vi "scada.vi"() -> ()   [LabVIEW 2014]
panel:
  in  "?":bool
  out "B7":bool
  out "B6":bool
  out "B5":bool
  out "B4":bool
  out "B2":bool
  out "B1":bool
  out "B3":bool
  out "Actuator 2 push L":bool
  out "Actuator 3 push L":bool
  out "Actuator 1 push R":bool
  out "Actuator 1 push L":bool
  in  "?":bool
  in  "?":bool
  in  "?":bool
  in  "?":bool
  in  "?":bool
  out "FAULT":bool
  out "RIGHT":bool
  out "CENTER":bool
  out "LEFT":bool
  out "ON/OFF":bool
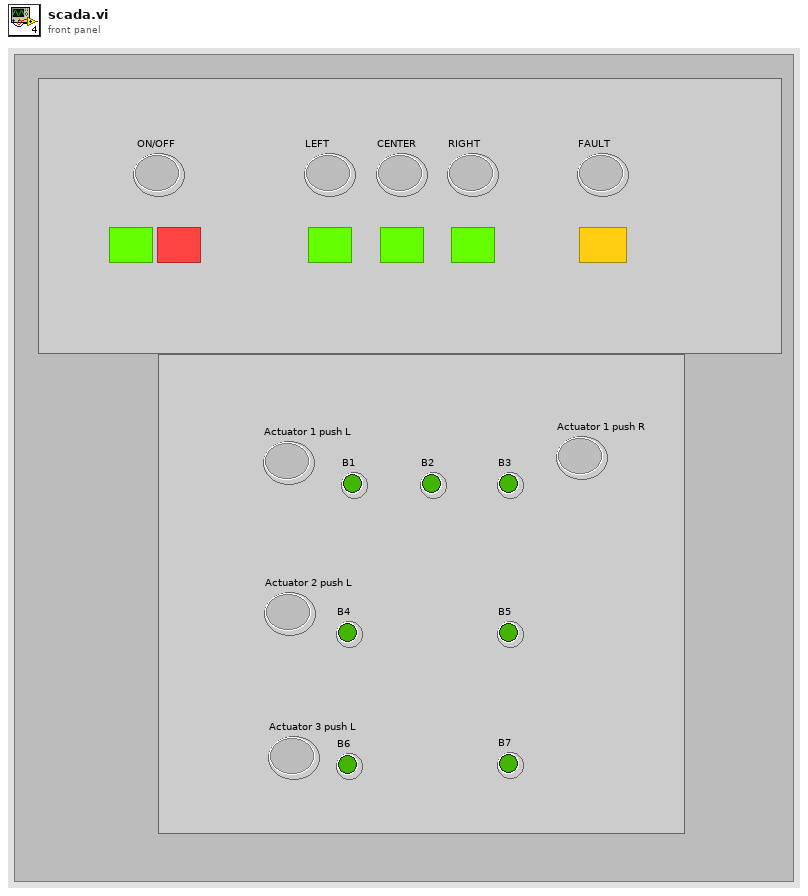
[diagram p1: front panel]
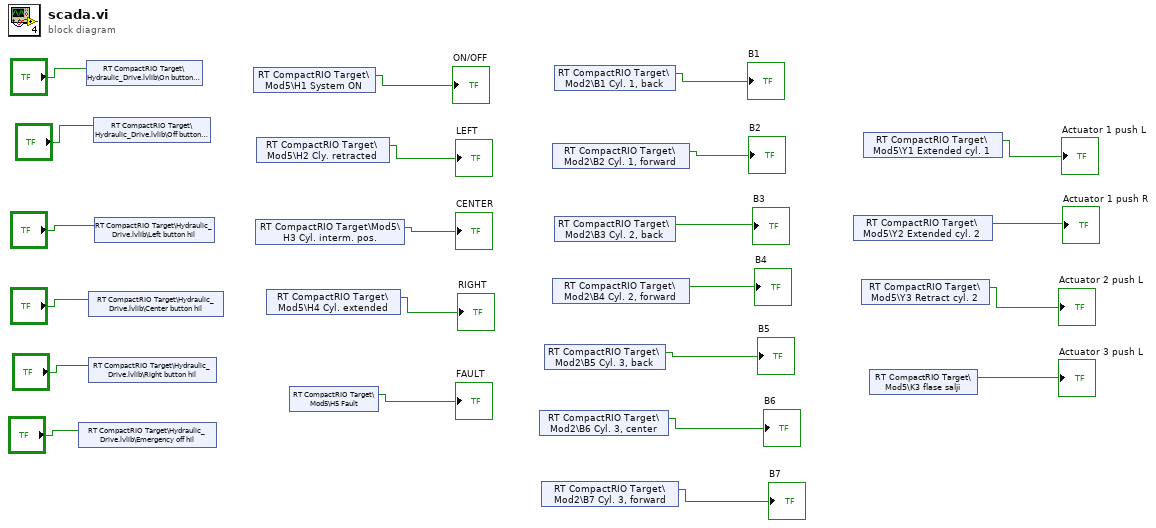
[diagram p0: block diagram]
diagram:
  n1 = shared-variable "RT CompactRIO Target\\Hydraulic_Drive.lvlib\\Emergency off hil"("?") -> ()  [unwired: 1 in, 1 out]
  n2 = shared-variable "RT CompactRIO Target\\Hydraulic_Drive.lvlib\\On button hil"("?") -> ()  [unwired: 1 in, 1 out]
  n3 = shared-variable "RT CompactRIO Target\\Hydraulic_Drive.lvlib\\Center button hil"("?") -> ()  [unwired: 1 in, 1 out]
  n4 = shared-variable "RT CompactRIO Target\\Hydraulic_Drive.lvlib\\Right button hil"("?") -> ()  [unwired: 1 in, 1 out]
  n5 = shared-variable "RT CompactRIO Target\\Hydraulic_Drive.lvlib\\Off button hil"("?") -> ()  [unwired: 1 in, 1 out]
  n6 = shared-variable "RT CompactRIO Target\\Hydraulic_Drive.lvlib\\Left button hil"("?") -> ()  [unwired: 1 in, 1 out]
  n7 = shared-variable "RT CompactRIO Target\\Mod5\\H1 System ON"() -> (→"ON/OFF":bool)  [unwired: 1 in, 1 out]
  n8 = shared-variable "RT CompactRIO Target\\Mod5\\H3 Cyl. interm. pos."() -> (→"CENTER":bool)  [unwired: 1 in, 1 out]
  n9 = shared-variable "RT CompactRIO Target\\Mod5\\H2 Cly. retracted"() -> (→"LEFT":bool)  [unwired: 1 in, 1 out]
  n10 = shared-variable "RT CompactRIO Target\\Mod5\\H4 Cyl. extended"() -> (→"RIGHT":bool)  [unwired: 1 in, 1 out]
  n11 = shared-variable "RT CompactRIO Target\\Mod5\\H5 Fault"() -> (→"FAULT":bool)  [unwired: 1 in, 1 out]
  n12 = shared-variable "RT CompactRIO Target\\Mod2\\B6 Cyl. 3, center"() -> (→"B6":bool)  [unwired: 1 in, 1 out]
  n13 = shared-variable "RT CompactRIO Target\\Mod2\\B7 Cyl. 3, forward"() -> (→"B7":bool)  [unwired: 1 in, 1 out]
  n14 = shared-variable "RT CompactRIO Target\\Mod2\\B5 Cyl. 3, back"() -> (→"B5":bool)  [unwired: 1 in, 1 out]
  n15 = shared-variable "RT CompactRIO Target\\Mod2\\B2 Cyl. 1, forward"() -> (→"B2":bool)  [unwired: 1 in, 1 out]
  n16 = shared-variable "RT CompactRIO Target\\Mod2\\B4 Cyl. 2, forward"() -> (→"B4":bool)  [unwired: 1 in, 1 out]
  n17 = shared-variable "RT CompactRIO Target\\Mod2\\B1 Cyl. 1, back"() -> (→"B1":bool)  [unwired: 1 in, 1 out]
  n18 = shared-variable "RT CompactRIO Target\\Mod2\\B3 Cyl. 2, back"() -> (→"B3":bool)  [unwired: 1 in, 1 out]
  n19 = shared-variable "RT CompactRIO Target\\Mod5\\Y2 Extended cyl. 2"() -> (→"Actuator 1 push R":bool)  [unwired: 1 in, 1 out]
  n20 = shared-variable "RT CompactRIO Target\\Mod5\\Y3 Retract cyl. 2"() -> (→"Actuator 2 push L":bool)  [unwired: 1 in, 1 out]
  n21 = shared-variable "RT CompactRIO Target\\Mod5\\Y1 Extended cyl. 1"() -> (→"Actuator 1 push L":bool)  [unwired: 1 in, 1 out]
  n22 = shared-variable "RT CompactRIO Target\\Mod5\\K3 flase salji"() -> (→"Actuator 3 push L":bool)  [unwired: 1 in, 1 out]
